vi "Actor Core.vi"(8 "error in":errorcluster, 11 "Nested in":refnum<class "Object Dictionary UI.lvclass">) -> (0 "error out":errorcluster, 3 "Actor out":refnum<class "Actor.lvclass">)   [LabVIEW 2020, in "Object Dictionary UI.lvlib" / "Object Dictionary UI.lvclass"]
doc: "(<B>Filename</B>: Actor Framework.lvlib:Actor.lvclass:Actor Core.vi)\n\nReceives messages to the actor, reacts to them, and initiates any error handling that may shut the actor down.\n\nDescendant classes may override this VI to append parallel tasks for the actor to complete while it handles messages. Overrides use the Call Parent Method node."
uses:
  Object Dictionary UI.lvclass
  Object Dictionary UI.lvclass/Object Dictionary UI.ctl
  <vilib>/ActorFramework/Stop Msg/Stop Msg.lvclass
  <vilib>/MGI/Panel Manager/Panel Actor/Panel Actor/Panel Actor.lvclass
  <vilib>/ActorFramework/Actor/Actor.lvclass
  Interactor Messages/Request OD Entry Values Msg/Request OD Entry Values Msg.lvclass
  Object Dictionary UI Messages/Populate Entry Details Msg/Populate Entry Details Msg.lvclass
  source/CANopen.lvlib
  Interactor Messages/Download OD Values Msg/Download OD Values Msg.lvclass
  <vilib>/Utility/miscctls.llb/LVRowAndColumnUnsignedTypeDef.ctl
  <vilib>/MGI/Panel Manager/Panel/Panel Helper/Events.ctl
  <vilib>/MGI/Panel Manager/Panel/Panel Helper/Panel Helper.lvclass
  <vilib>/MGI/Panel Manager/Panel/Panel Helper/Panel Events.ctl
  source/Typedefs/Object Type.ctl
  source/Typedefs/Access SDO.ctl
  source/Typedefs/Access PDO.ctl
  source/Typedefs/Access SRDO.ctl
  EDS-File-Viewer/source/UI Actor/Controls/Object Details.ctl
  EDS-File-Viewer/source/UI Actor/UI Actor/UI Actor.lvclass
  source/Typedefs/Access Type.ctl
  source/Typedefs/Data Type.ctl
  EDS-File-Viewer/source/UI Actor/Controls/Sub Objects Table Entry.ctl
panel:
  out "Sub Objects Table":T1[](array[typedef]) {"Sub Index" format="%02x"; "Data Type" items=["unknown", "BOOLEAN", "INTEGER8", "INTEGER16", "INTEGER32", "UNSIGNED8", "UNSIGNED16", "UNSIGNED32", "REAL32", "VISIBLE_STRING", "OCTET_STRING", "UNICODE_STRING", "TIME_OF_DAY", "TIME_DIFFERENCE", "RESERVED1", "DOMAIN", "INTEGER24", "REAL64", "INTEGER40", "INTEGER48", "INTEGER56", "INTEGER64", "UNSIGNED24", "RESERVED2", "UNSIGNED40", "UNSIGNED48", "UNSIGNED56", "UNSIGNED64", "RESERVED3", "RESERVED4", "RESERVED5", "RESERVED6", "PDO_COMMUNICATION_PARAMETER", "PDO_MAPPING", "SDO_PARAMETER", "IDENTITY", "RESERVED7"]}
  in  "Object Details":T4 {"Data Type" items=["unknown", "BOOLEAN", "INTEGER8", "INTEGER16", "INTEGER32", "UNSIGNED8", "UNSIGNED16", "UNSIGNED32", "REAL32", "VISIBLE_STRING", "OCTET_STRING", "UNICODE_STRING", "TIME_OF_DAY", "TIME_DIFFERENCE", "RESERVED1", "DOMAIN", "INTEGER24", "REAL64", "INTEGER40", "INTEGER48", "INTEGER56", "INTEGER64", "UNSIGNED24", "RESERVED2", "UNSIGNED40", "UNSIGNED48", "UNSIGNED56", "UNSIGNED64", "RESERVED3", "RESERVED4", "RESERVED5", "RESERVED6", "PDO_COMMUNICATION_PARAMETER", "PDO_MAPPING", "SDO_PARAMETER", "IDENTITY", "RESERVED7"]; "ObjectType" items=["NULL"=0, "DOMAIN"=2, "DEFTYPE"=5, "DEFSTRUCT"=6, "VAR"=7, "ARRAY"=8, "RECORD"=9]; "Sub Index" format="%02x"; "Index" format="%04x"}
  out "Device Profile Specific":cluster{"Index":u16, "Name":string}[](array[cluster]) {"Index" format="%04x"}
  out "Manufacturer Specific":cluster{"Index":u16, "Name":string}[](array[cluster]) {"Index" format="%04x"}
  out "Communication Profile":cluster{"Index":u16, "Name":string}[](array[cluster]) {"Index" format="%04x"}
  # "Sub Idx"
  # "Name"
  # "Data Type"
  # "SDO"
  # "PDO"
  # "Default Value"
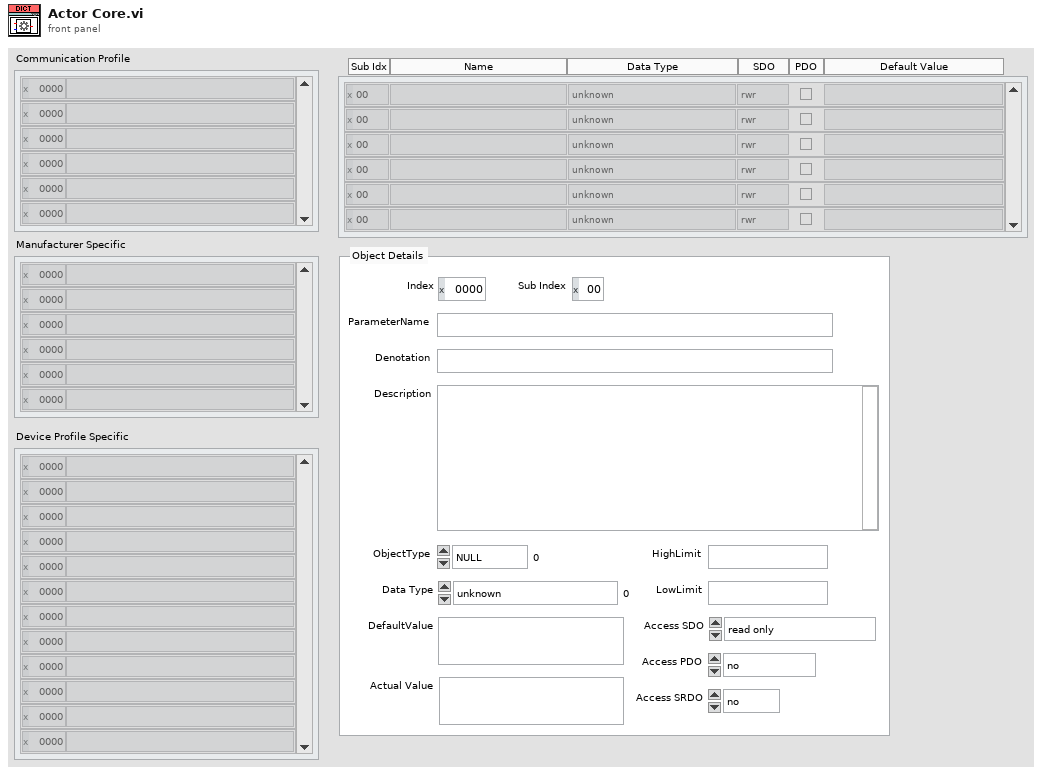
[diagram p1: front panel]
types:
  T1 = typedef "UI Actor.lvlib/UI Actor.lvclass/Sub Objects Table Entry.ctl" = cluster{"Sub Index":u8, "Name":string, "Data Type":T2, "Access Type":T3, "PDO Mapping":bool, "Default Value":string}
  T2 = typedef "CANopen.lvlib/Data Type.ctl" = u16
  T3 = typedef "CANopen.lvlib/Access Type.ctl" = enum16{"unknown", "ro", "wo", "rw", "rwr", "rww", "const"}
  T4 = typedef "UI Actor.lvlib/UI Actor.lvclass/Object Details.ctl" = cluster{"Denotation":string, "Description":string, "ParameterName":string, "Index":u16, "Sub Index":u8, "ObjectType":T5, "Data Type":u16, "HighLimit":string, "LowLimit":string, "Access SDO":T6, "Access PDO":T7, "Access SRDO":T8, "Actual Value":string, "DefaultValue":string}
  T5 = typedef "CANopen.lvlib/Object Type.ctl" = u8
  T6 = typedef "CANopen.lvlib/Access SDO.ctl" = enum16{"read only", "write only", "read/write", "read/write on process input", "read/write on process output", "constant value", "no", "UNKNOWN"}
  T7 = typedef "CANopen.lvlib/Access PDO.ctl" = enum16{"no", "TPDO", "RPDO", "TPDO & RPDO"}
  T8 = typedef "CANopen.lvlib/Access SRDO.ctl" = enum16{"no", "tx", "rx", "trx"}
  T9 = cluster{"Pnl Actor":refnum<event-registration>, "Custom":refnum<event-registration>}
  T10 = typedef "LVRowAndColumnUnsignedTypeDef.ctl" = cluster{"Row":u32, "Column":u32}
  T11 = enum8{"Enabled", "Disabled", "Disabled and Grayed Out"}
  T12 = cluster{"Communication Specific Objects":refnum<user-event>, "Attribute Table":refnum<user-event>, "Entry Details":refnum<user-event>}
  T13 = cluster{"Multiplexer":cluster{"Index":u16, "Sub-Index":i16}, "Value":variant}
  T14 = typedef "LVRowAndColumnTypeDef.ctl" = cluster{"Row":i32, "Column":i32}
  T15 = cluster{"Multiplexer":cluster{"Index":u16, "Sub-Index":i16}, "Value":variant}[]
  T16 = typedef "LVPoint32TypeDef.ctl" = cluster{"Horizontal":i32, "Vertical":i32}
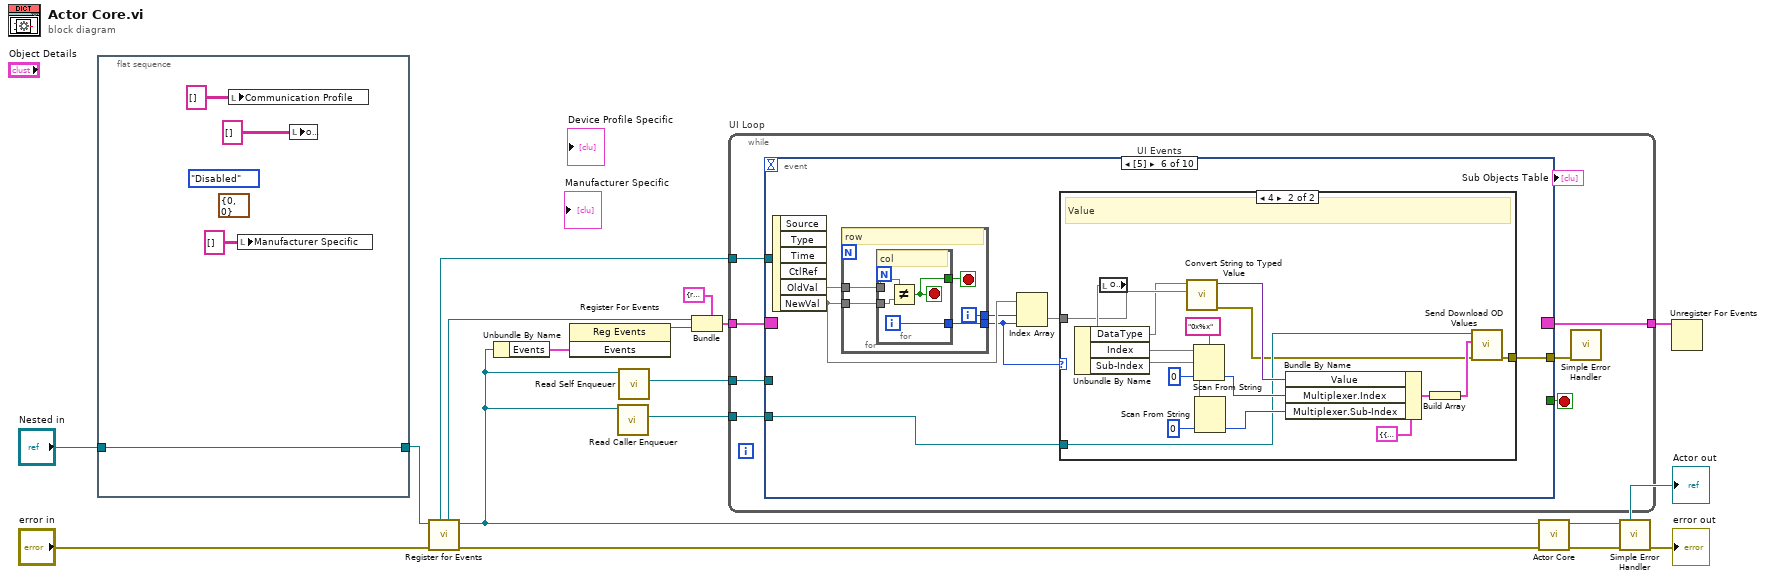
[diagram p0: block diagram]
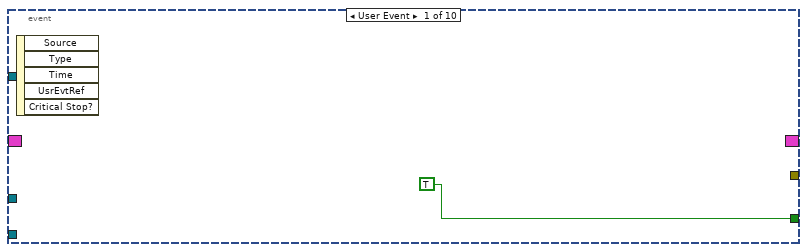
[diagram p2: hidden frame]
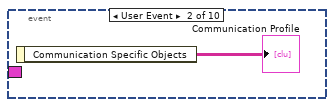
[diagram p3: hidden frame]
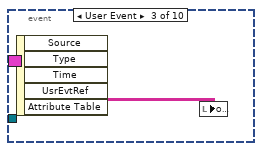
[diagram p4: hidden frame]
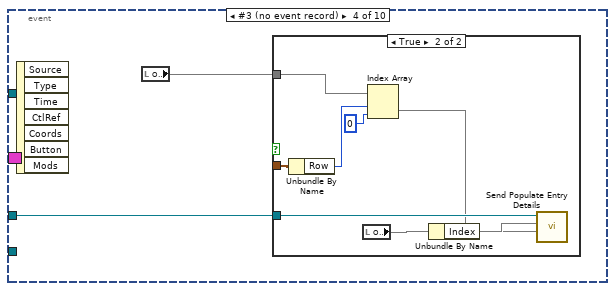
[diagram p5: hidden frame]
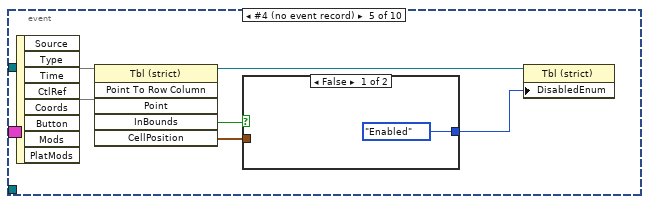
[diagram p7: hidden frame]
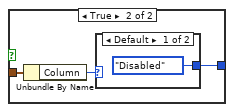
[diagram p8: hidden frame]
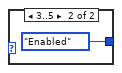
[diagram p9: hidden frame]
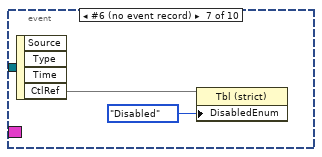
[diagram p11: hidden frame]
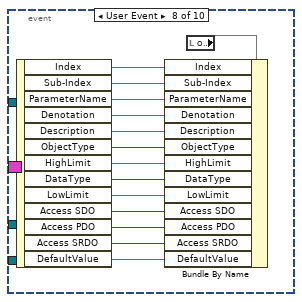
[diagram p12: hidden frame]
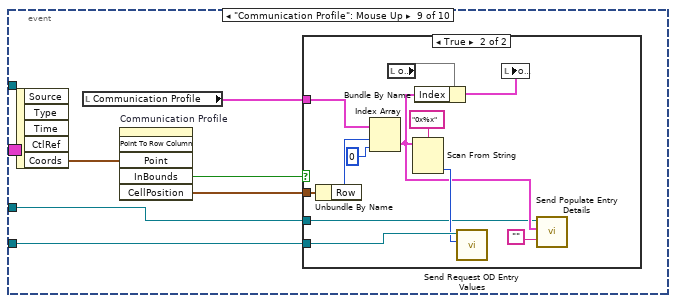
[diagram p13: hidden frame]
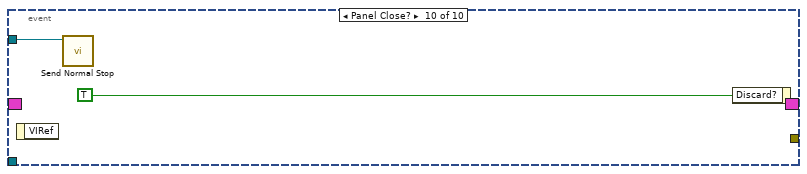
[diagram p15: hidden frame]
diagram:
  n1 = flat-sequence {
    tunnel: "Nested in" -> [w23]
    tunnel: [w23] -> w7
    frame #0 {
      w19 = T10 {"Row"=0, "Column"=0} ("Index Values")
      w20 = T11."Disabled" ("Disabled")
      n2 = local write "Communication Profile"(string[][] [] ("Communication Specific")) -> ()
      n3 = local write "Manufacturer Specific"(string[][] [] ("Manufacturer Specific")) -> ()
      n4 = local write item#-1(string[][] [] ("Attribute Table")) -> ()
    }
  }
  n5 = call <vilib>:"Register for Events.vi"("Error In"="error in", "Panel Actor in"=w7) -> ("Error Out"=w9:errorcluster, "Panel Actor out"=w3:refnum<class "Object Dictionary UI.lvclass">, "Pnl Actor"=w10:refnum<event-registration>, "Self Enqueuer"=w12:refnum<class "Message Enqueuer.lvclass">)  [unwired: 6 in]
  n6 = Unbundle By Name(w3) -> ("Events"=w15:T12)
  n7 = register-events ("Main Register for Events")(w15) -> (reference out=w5:refnum<event-registration>)  [unwired: 2 in, 1 out]
  n8 = call <vilib>:"Read Caller Enqueuer.vi"("Actor"=w3) -> ("Caller Enqueuer"=w6:refnum<class "Message Enqueuer.lvclass">)  [unwired: 10 in]
  n9 = call <vilib>:"Read Self Enqueuer.vi"("Actor"=w3) -> ("Self Enqueuer"=w2:refnum<class "Message Enqueuer.lvclass">)  [unwired: 10 in]
  n10 = Bundle(cluster=T9 {"Pnl Actor"=refnum, "Custom"=refnum}, "Pnl Actor"=w10, "Custom"=w5) -> (w11:T9)
  n11 = while "UI Loop" {
    tunnel: w11 -> [w30]
    tunnel: [w28] -> w14
    tunnel: w12 -> [w27]
    tunnel: w6 -> [w26]
    tunnel: w2 -> [w25]
    stop <- w29 stop-if-true
    n12 = event "UI Events" shown="[5]" {
      selector: w30 -> [_ _ _ _ _ _ _ _ _ _]
      dyn-events: [_ _ _ _ _ _ _ _ _ _] -> w28
      timeout: _ -> [_ _ _ _ _ _ _ _ _ _]
      tunnel: [TRUE _ _ _ _ _ _ _ _ _] -> w29
      tunnel: w27 -> [_ _ _ _ _ _ _ _ _ w127]
      tunnel: w26 -> [_ _ _ _ _ w59 _ _ w111 _]
      tunnel: w25 -> [_ _ _ w34 _ _ _ _ w109 _]
      tunnel: [_ _ _ _ _ w60 _ _ _ _] -> w24
      event User Event {
        n13 = event-data() -> ()  [unwired: 1 in, 5 out]
      }
      event User Event {
        n14 = event-data() -> ("Communication Specific Objects"=→"Communication Profile":string[][])  [unwired: 1 in]
      }
      event User Event {
        n15 = event-data() -> ("Attribute Table"=w33:string[][])  [unwired: 1 in, 4 out]
        n16 = local write item#-1(w33) -> ()
      }
      event #3 (no event record) {
        n17 = event-data() -> ("Coords"=w38)  [unwired: 1 in, 6 out]
        n18 = local read item#-1() -> (w35)
        n19 = case shown="True" w37 {
          tunnel: [_ w46] -> w36
          tunnel: w35 -> [_ w44]
          tunnel: w34 -> [_ w42]
          frame False {
          }
          frame True {
            n20 = Unbundle By Name(w46) -> ("Row"=w43:i32)
            n21 = local read item#-1() -> (w41)
            n22 = Index Array(array=w44, index (row)=w43, index (col)=0) -> (element=w39)
            n23 = Unbundle By Name(w41) -> ("Index"=w40)
            n24 = call "Send Populate Entry Details.vi"("Sub-Index"=w39, "Index"=w40, "Message Enqueuer"=w42) -> ()  [unwired: 7 in, 2 out]
          }
        }
      }
      event #4 (no event record) {
        n25 = event-data() -> ("CtlRef"=w48, "Coords"=w49)  [unwired: 1 in, 6 out]
        n26 = invoke class="Tbl (strict)" method="Point To Row Column"(reference=w48, "Point"=w49) -> (reference out=w50:refnum<vi>, "InBounds"=w52:bool, "CellPosition"=w51:T14)  [unwired: 4 in, 3 out]
        n27 = case shown="False" w52 {
          tunnel: w51 -> [_ w56]
          tunnel: [T11."Enabled" ("Disabled") w54] -> w47
          frame False {
          }
          frame True {
            n28 = Unbundle By Name(w56) -> ("Column"=w55:i32)
            n29 = case shown="Default" w55 {
              tunnel: [T11."Disabled" ("Disabled") T11."Enabled" ("Disabled")] -> w54
              frame Default {
              }
              frame 3..5 {
              }
            }
          }
        }
        n30 = property class="Tbl (strict)"(reference=w50, "DisabledEnum"=w47) -> ()  [unwired: 1 in, 2 out]
      }
      event #5 (no event record) {
        n31 = event-data() -> ("OldVal"=w65, "NewVal"=w64)  [unwired: 1 in, 4 out]
        n32 = for {
          tunnel: w65 -> [w70]
          tunnel: w64 -> [w69]
          tunnel: [w68] -> w62
          tunnel: [w67] -> w63
          i -> [w67]
          stop <- w66 stop-if-true
          # "row"
          n33 = for {
            tunnel: w70 -> [w74]
            tunnel: w69 -> [w73]
            tunnel: [w72] -> w68
            tunnel: [w71] -> w66
            i -> [w72]
            stop <- w71 stop-if-true
            # "col"
            n34 = Not Equal?(x=w74, y=w73) -> (x != y?=w71:bool)
          }
        }
        n35 = Index Array(array=w64, index (row)=w63, index (col)=w62) -> (element=w61)
        n36 = case shown="4" w62 {
          tunnel: w61 -> [_ w90]
          tunnel: [_ w76] -> w60
          tunnel: w59 -> [_ w78]
          frame 0, Default {
          }
          frame 4 {
            # "Value"
            n37 = local read item#-1() -> (w91)
            n38 = Unbundle By Name(w91) -> ("DataType"=w89, "Index"=w84, "Sub-Index"=w79)
            n39 = call "Convert String to Typed Value.vi"("Value"=w90, "DataType"=w89) -> ("error out"=w77:errorcluster, "Typed Value"=w87:variant)  [unwired: 8 in]
            n40 = Scan From String(format string="0x%x", input string=w84, default 1=u16 0 ("Multiplexer.Index")) -> (output 1=w83:u16)  [unwired: 2 in, 3 out]
            n41 = Scan From String(input string=w79, default 1=i16 0 ("Multiplexer.Sub-Index")) -> (output 1=w80:i16)  [unwired: 3 in, 3 out]
            n42 = Bundle By Name(cluster=T13 {"Multiplexer"={"Index"=0, "Sub-Index"=0}, "Value"=variant}, "Value"=w87, "Multiplexer.Index"=w83, "Multiplexer.Sub-Index"=w80) -> (w85:T13)
            n43 = Build Array(w85) -> (w86:T15)
            n44 = call "Send Download OD Values.vi"("error in (no error)"=w77, "Values"=w86, "Message Enqueuer"=w78) -> ("error out"=w76:errorcluster)  [unwired: 7 in, 1 out]
          }
        }
      }
      event #6 (no event record) {
        n45 = event-data() -> ("CtlRef"=w93)  [unwired: 1 in, 3 out]
        n46 = property class="Tbl (strict)"(reference=w93, "DisabledEnum"=T11."Disabled" ("Disabled")) -> ()  [unwired: 1 in, 2 out]
      }
      event User Event {
        n47 = event-data() -> ("Index"=w107:string, "Sub-Index"=w106:string, "ParameterName"=w105:string, "Denotation"=w104:string, "Description"=w103:string, "ObjectType"=w102:T5, "HighLimit"=w101:string, "DataType"=w100:u16, "LowLimit"=w99:string, "Access SDO"=w98:T6, "Access PDO"=w97:T7, "Access SRDO"=w96:T8, "DefaultValue"=w95:string)  [unwired: 1 in]
        n48 = local read item#-1() -> (w108)
        n49 = Bundle By Name(cluster=w108, "Index"=w107, "Sub-Index"=w106, "ParameterName"=w105, "Denotation"=w104, "Description"=w103, "ObjectType"=w102, "HighLimit"=w101, "DataType"=w100, "LowLimit"=w99, "Access SDO"=w98, "Access PDO"=w97, "Access SRDO"=w96, "DefaultValue"=w95) -> (w94:cluster{})
      }
      event "Communication Profile": Mouse Up {
        n50 = event-data() -> ("Coords"=w114:T16)  [unwired: 1 in, 4 out]
        n51 = local read "Communication Profile"() -> (w112:cluster{"Index":u16, "Name":string}[])
        n52 = invoke on="Communication Profile" class="Arr (strict)" method="Point To Row Column"("Point"=w114) -> ("InBounds"=w110:bool, "CellPosition"=w113:T14)  [unwired: 5 in, 4 out]
        n53 = case shown="True" w110 {
          tunnel: w113 -> [_ w126]
          tunnel: w112 -> [_ w125]
          tunnel: w111 -> [_ w121]
          tunnel: w109 -> [_ w115]
          frame False {
          }
          frame True {
            n54 = Unbundle By Name(w126) -> ("Row"=w124:i32)
            n55 = Index Array(array=w125, index (row)=w124, index (col)=0) -> (element=w117:cluster{"Index":u16, "Name":string})
            n56 = local read item#-1() -> (w119)
            n57 = Scan From String(format string="0x%x", input string=w117) -> (output 1=w120:u16)  [unwired: 3 in, 3 out]
            n58 = Bundle By Name(cluster=w119, "Index"=w117) -> (w118:cluster{})
            n59 = call "Send Request OD Entry Values.vi"("Index"=w120, "Message Enqueuer"=w121) -> ()  [unwired: 8 in, 2 out]
            n60 = local write item#-1(w118) -> ()
            n61 = call "Send Populate Entry Details.vi"("Sub-Index"="", "Index"=w117, "Message Enqueuer"=w115) -> ()  [unwired: 7 in, 2 out]
          }
        }
      }
      event Panel Close? {
        n62 = event-data() -> ()  [unwired: 1 in, 1 out]
        n63 = call <vilib>:"Send Normal Stop.vi"("Message Enqueuer"=w127) -> ()  [unwired: 10 in, 1 out]
        n64 = event-data("Discard?"=TRUE) -> ()  [unwired: 1 in, 1 out]
      }
    }
    n65 = call <vilib>:"Simple Error Handler.vi"("error in (no error)"=w24) -> ()  [unwired: 4 in, 5 out]
  }
  n66 = call-parent "Actor Core.vi"("error in"=w9, "Panel Actor in"=w3) -> ("error out"=w17:errorcluster, "Actor out"=→"Actor out":refnum<class "Actor.lvclass">)  [unwired: 8 in]
  n67 = call <vilib>:"Simple Error Handler.vi"("error in (no error)"=w17) -> ("error out"=→"error out":errorcluster)  [unwired: 4 in, 4 out]
  n68 = Unregister For Events(event registration refnum=w14) -> ()  [unwired: 1 in, 1 out]
